vi "Update Result Name.vi"(7 "LV Result Name Property":string, 8 "error in (no error)":errorcluster, 10 "Step In":refnum<k7>, 11 "SPECAN_PVT in":refnum<class "SPECAN_PVT.lvclass">) -> (0 "error out":errorcluster, 2 "Step Out":refnum<k7>, 3 "SPECAN_PVT out":refnum<class "SPECAN_PVT.lvclass">)   [LabVIEW 2018, in "SPECAN_PVT.lvlib" / "SPECAN_PVT.lvclass"]
uses:
  SPECAN_PVT.lvclass
  SPECAN_PVT.lvclass/SPECAN_PVT.ctl
  Read Result Name.vi
  Plugins/TestStand API Tools (TSAT).lvlibp/Step Actions/TSAT Step Actions.lvlib
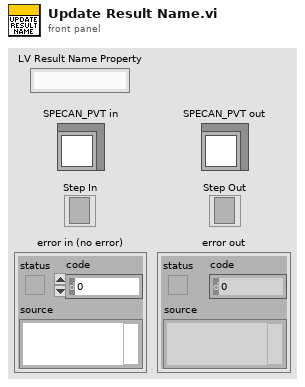
[diagram p1: front panel]
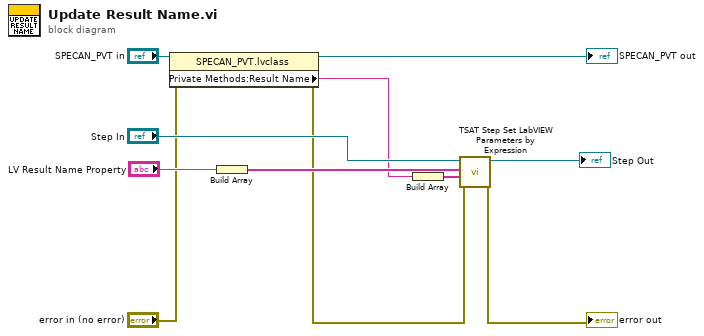
[diagram p0: block diagram]
diagram:
  n1 = property class="SPECAN_PVT.lvclass"(reference="SPECAN_PVT in", error in="error in (no error)") -> (reference out=→"SPECAN_PVT out":refnum<class "SPECAN_PVT.lvclass">, error out=w3:errorcluster, "Private Methods:Result Name"=w6:string)
  n2 = Build Array("LV Result Name Property") -> (w8:string[])
  n3 = Build Array(w6) -> (w5:string[])
  n4 = call "TSAT Step Set LabVIEW Parameters by Expression.vi"("Error In"=w3, "Value Expressions"=w5, "Parameters to Set"=w8, "Step In"="Step In") -> ("Error Out"=→"error out":errorcluster, "Step Out"=→"Step Out":refnum<k7>)  [unwired: 6 in]
